vi "Configure Output Enable.vi"(8 "error in (no error)":errorcluster, 9 "enabled (true)":bool=TRUE, 10 "channel name (\"CHANNEL1\")":string="CHANNEL1", 11 "CS++DCPwr in":refnum<class "CS++DCPwr.lvclass">) -> (0 "error out":errorcluster, 3 "CS++DCPwr out":refnum<class "CS++DCPwr.lvclass">)   [LabVIEW 2013, in "CS++DCPwr.lvlib" / "CS++DCPwr.lvclass"]
doc: "Configures whether the signal that the power supply produces on a channel appears at the output connector."
uses:
  CS++DCPwr.lvclass
  Core/Classes/CS++ProcessVariables/ProcessVariable/PV.lvclass
  Core/Classes/CS++ProcessVariables/ProcessVariable/PV.lvclass/PV.ctl
  CS++DCPwr.lvclass/CS++DCPwr.ctl
  Core/Classes/CS++ProcessVariables/PVConnection/PVConnection.lvclass
  Core/Classes/CS++ProcessVariables/ProcessVariable/Write Data.vi
  Core/Classes/CS++ProcessVariables/ProcessVariable/Write Timestamp.vi
  Core/Classes/CS++ProcessVariables/ProcessVariable/Write Quality.vi
  Core/Classes/CS++ProcessVariables/ProcessVariable/Write status.vi
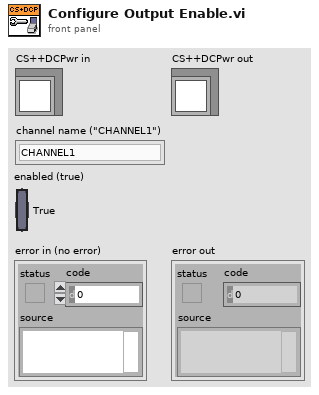
[diagram p1: front panel]
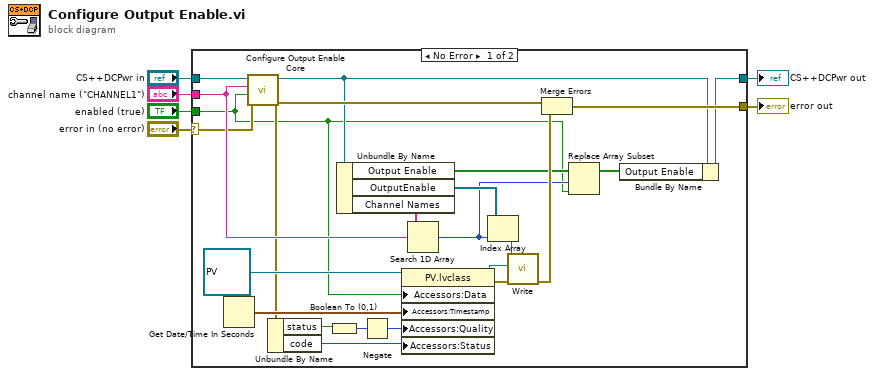
[diagram p0: block diagram]
diagram:
  n1 = case shown="No Error" "error in (no error)" {
    selector: "error in (no error)" -> [w8 w30]
    tunnel: "CS++DCPwr in" -> [w29 w31]
    tunnel: "enabled (true)" -> [w7 _]
    tunnel: "channel name (\"CHANNEL1\")" -> [w16 _]
    tunnel: [w14 w30] -> w2
    tunnel: [w12 w31] -> w1
    frame No Error {
      n2 = Get Date/Time In Seconds() -> (seconds since 1Jan1904=w28:timestamp)
      n3 = call-dynamic "Configure Output Enable Core.vi"("error in (no error)"=w8, "enabled (true)"=w7, "channel name (\"CHANNEL1\")"=w16, "CS++DCPwr in"=w29) -> ("error out"=w15:errorcluster, "CS++DCPwr out"=w13:refnum<class "CS++DCPwr.lvclass">)  [unwired: 6 in]
      n4 = Unbundle By Name(w15) -> ("status"=w20:bool, "code"=w18:i32)
      n5 = Boolean To (0,1)(Boolean=w20) -> (0, 1=w19:i16)
      n6 = Unbundle By Name(w13) -> ("Output Enable"=w11:bool[], "OutputEnable"=w23:refnum<class "PVConnection.lvclass">[], "Channel Names"=w24:string[])
      n7 = Negate(x=w19) -> (-x=w17:i16)
      n8 = property class="PV.lvclass"(reference=refnum<class "PV.lvclass"> refnum ("PV"), "Accessors:Data"=w7, "Accessors:Timestamp"=w28, "Accessors:Quality"=w17, "Accessors:Status"=w18) -> (reference out=w25:refnum<class "PV.lvclass">, error out=w26:errorcluster)  [unwired: 1 in]
      n9 = Search 1D Array(1D array=w24, element=w16) -> (index of element=w9:i32)  [unwired: 1 in]
      n10 = Index Array(array=w23, index=w9) -> (element=w22:refnum<class "PVConnection.lvclass">)
      n11 = call-dynamic "Write.vi"("error in (no error)"=w26, "PV"=w25, "PVConnection in"=w22) -> ("error out"=w21:errorcluster)  [unwired: 7 in, 1 out]
      n12 = Merge Errors(w15, w21) -> (w14:errorcluster)
      n13 = Replace Array Subset(array=w11, new element=w7, index=w9) -> (w10:bool[])
      n14 = Bundle By Name(cluster=w13, "Output Enable"=w10) -> (w12:refnum<class "CS++DCPwr.lvclass">)
    }
    frame Error {
    }
  }
  "error out" <- w2
  "CS++DCPwr out" <- w1
